vi "CopyServerCode.vi"() -> ()   [LabVIEW 2019]
uses:
  <vilib>/Utility/traverseref.llb/VI Scripting - Traverse.lvlib
  <vilib>/Utility/traverseref.llb/TRef TravTarget.ctl
  <vilib>/Utility/miscctls.llb/LVPositionTypeDef.ctl
panel:
  out "Backup path":path
  out "error out":errorcluster
  in  "Destination server name":string="gRPC1.6_Template2_server"
  in  "Source server name":string="gRPC1.6_Template_server"
  in  "target name":string="My Computer"
  in  "Project path":path=path "D:/temp test/gRPC1.6_Template.lvproj"
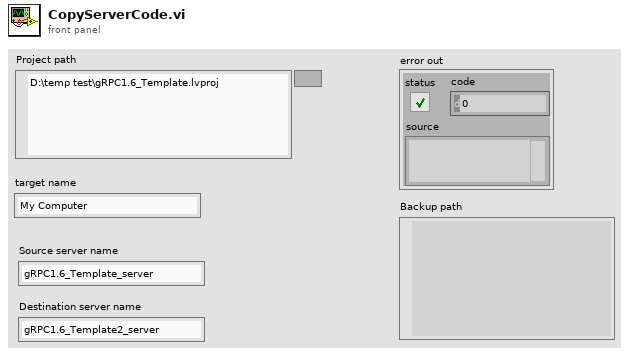
[diagram p1: front panel]
types:
  T1 = cluster{"dest":refnum<vi>, "source":refnum<vi>}[]
  T2 = cluster{"DstDiagram":refnum<vi>, "DestIndex":i32, "DstEvntStr":refnum<vi>, "SrcDiagram":refnum<vi>, "SrcIndex":i32, "SrcEvntStr":refnum<vi>}[]
  T3 = cluster{"ClassName":string, "Dest_SyncRef":refnum<vi>, "Dest_AsyncRef":refnum<vi>, "Source_SyncRef":refnum<vi>, "Source_AsyncRef":refnum<vi>}[]
  T4 = cluster{"Name":string, "DestRef":refnum<vi>, "SourceRef":refnum<vi>}[]
  T5 = cluster{string, "DestRef":refnum<vi>, refnum<vi>}
  T6 = cluster{"Name":string, "Dest_SyncRef":refnum<vi>, "Dest_AsyncRef":refnum<vi>, "Source_SyncRef":refnum<vi>, "Source_AsyncRef":refnum<vi>}
  T7 = cluster{"Name":string, "Dest_SyncRef":refnum<vi>, "Dest_AsyncRef":refnum<vi>, "Source_SyncRef":refnum<vi>, "Source_AsyncRef":refnum<vi>}[]
  T8 = typedef "TRef TravTarget.ctl" = enum16{"FP", "BD", "Other"}
  T9 = cluster{"Dest_SyncRef":refnum<vi>, "Source_SyncRef":refnum<vi>}
  T10 = cluster{"VI Ref":refnum<vi>, "VI Ref":refnum<vi>}
  T11 = cluster{"VI Ref":refnum<vi>, "VI Ref":refnum<vi>}[]
  T12 = cluster{refnum<vi>, "index of element":i32, refnum<vi>, refnum<vi>, i32, refnum<vi>}
  T13 = cluster{"DstDiagram":refnum<vi>, "index of element":i32, "DstEvntStr":refnum<vi>, "SrcDiagram":refnum<vi>, "SrcIndex":i32, "SrcEvntStr":refnum<vi>}[]
  T14 = typedef "LVPositionTypeDef.ctl" = cluster{"Left":i32, "Top":i32}
  T15 = cluster{"Src Name":string, "VI Name":string, "VI Term Name":string}[]
  T16 = cluster{"Src Name":string, "VIName":string, "Name":string}[]
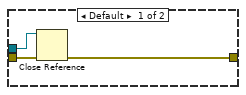
[diagram p4: hidden frame]
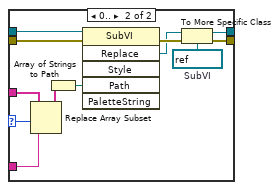
[diagram p5: hidden frame]
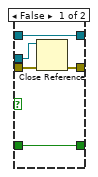
[diagram p8: hidden frame]
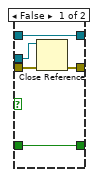
[diagram p9: hidden frame]
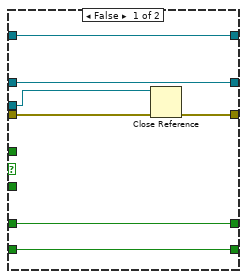
[diagram p10: hidden frame]
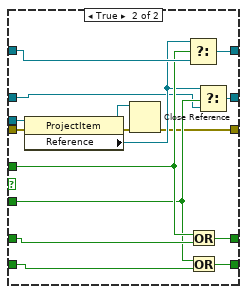
[diagram p11: hidden frame]
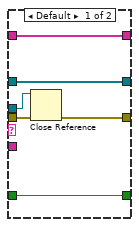
[diagram p12: hidden frame]
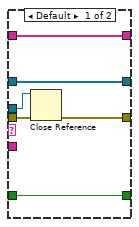
[diagram p13: hidden frame]
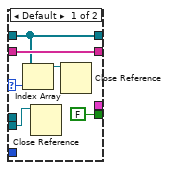
[diagram p14: hidden frame]
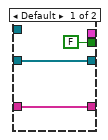
[diagram p15: hidden frame]
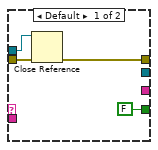
[diagram p16: hidden frame]
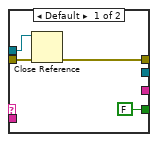
[diagram p17: hidden frame]
diagram:
  w22 = refnum<vi> refnum  # Library
  w18 = "Data Converters"
  w105 = "Backup_"
  w120 = T4 []  # CommonClasses
  w131 = string[] []  # SourceClassNames
  w129 = refnum<vi>[] []  # SourceClassPrjctRefs
  w132 = string[] []  # DestClassNames
  w136 = refnum<vi>[] []  # DestClassPrjctRefs
  w141 = refnum<vi> refnum  # Library
  w149 = refnum<vi> refnum  # Library
  w153 = ".lvlib"
  w157 = refnum<vi> refnum  # Source folder
  w158 = refnum<vi> refnum  # Dest folder
  w159 = FALSE  # found dest
  w160 = FALSE  # found source
  # "Copy destination library to source location\nand delete original destination."
  # "Verify and close project"
  # "Create Folder and add converter VIs"
  # "Add destination\nlibrary to new source\nfolder in project"
  # "Create new\nsource folder"
  # "Delete destination\nfolder\nfrom project"
  # "Delete source\ndirectory\nfrom disk"
  # "Delete source\ndirectory\nfrom project"
  # "Delete source\nlvlib from project"
  # "TODO:\nAdd check\nfor good name"
  n1 = Temporary Directory() -> (w78:path)
  n2 = Build Path(base path=w78, name or relative path=path "ServerBackups") -> (appended path=w76:path)
  n3 = Strip Path(path="Project path") -> (stripped path=w34:path)  [unwired: 1 out]
  n4 = List Folder(path=w34) -> (path out=w110:path, filenames=w139:string[], folder names=w107:string[])  [unwired: 3 in, 1 out]
  n5 = Create Folder(path (use dialog)=w76) -> (created path=w75:path)  [unwired: 2 in, 2 out]
  n6 = while {
    tunnel: w75 -> [w177]
    tunnel: [w172] -> w74
    tunnel: w105 -> [w171]
    i -> [w176]
    stop <- w173 continue-if-true
    # "Find Available\nBackup Directory"
    n7 = Number To Decimal String(number=w176) -> (decimal integer string=w174:string)  [unwired: 1 in]
    n8 = Concatenate Strings(w171, w174) -> (w175:string)
    n9 = Build Path(base path=w177, name or relative path=w175) -> (appended path=w172:path)
    n10 = call <vilib>:"Check if File or Folder Exists.vi"("path"=w172) -> ("file or folder exists?"=w173:bool)  [unwired: 8 in, 2 out]
  }
  "Backup path" <- w74
  n11 = Create Folder(path (use dialog)=w74) -> (created path=w109:path, error out=w140:errorcluster)  [unwired: 2 in, 1 out]
  n12 = for {
    shift-right: [w183] -> w108
    shift-left: w140 -> [w184]
    tunnel: w109 -> [w179]
    tunnel: w110 -> [w182]
    tunnel: w139 -> [w178] mode=indexing
    # "Backup Files"
    n13 = Build Path(base path=w182, name or relative path=w178) -> (appended path=w181:path)
    n14 = Build Path(base path=w179, name or relative path=w178) -> (appended path=w180:path)
    n15 = Copy(8:w184, 10:w180, 11:w181) -> (0:w183:errorcluster)  [unwired: 2 in, 2 out]
  }
  n16 = Concatenate Strings("^" ("string"), w105) -> (w104:string)
  n17 = for {
    shift-right: [w190] -> w7
    shift-left: w108 -> [w191]
    tunnel: w109 -> [w188]
    tunnel: w110 -> [w189]
    tunnel: w107 -> [w187] mode=indexing
    tunnel: w104 -> [w186]
    # "Backup Directories"
    n18 = Match Pattern(string=w187, regular expression=w186) -> (match substring=w185:string)  [unwired: 1 in, 3 out]
    n19 = case shown="Default" w185 {
      tunnel: w191 -> [w192 w199]
      tunnel: [w192 w198] -> w190
      tunnel: w189 -> [_ w197]
      tunnel: w188 -> [_ w194]
      tunnel: w187 -> [_ w193]
      frame "Backup_" {
        # "Don't backup\nprevious\nbackups"
      }
      frame Default {
        n20 = Build Path(base path=w197, name or relative path=w193) -> (appended path=w196:path)
        n21 = Build Path(base path=w194, name or relative path=w193) -> (appended path=w195:path)
        n22 = Copy(8:w199, 10:w195, 11:w196) -> (0:w198:errorcluster)  [unwired: 2 in, 2 out]
      }
    }
  }
  n23 = invoke class="App" method="Project.Open"(error in=w7, "Path"="Project path") -> (error out=w5:errorcluster, "Project:Open"=w6:refnum<vi>)  [unwired: 2 in, 2 out]
  n24 = invoke class="Project" method="Save"(reference=w6, error in=w5) -> (reference out=w2:refnum<vi>, error out=w3:errorcluster)  [unwired: 2 in, 2 out]
  n25 = Close Reference(reference=w2, error in (no error)=w3) -> (error out=w1:errorcluster)
  n26 = local read "Destination server name"() -> (w19:string)
  n27 = local read "Source server name"() -> (w32:string)
  n28 = Concatenate Strings(w19, ".lvlib" ("string")) -> (w27:string)
  n29 = Build Path(base path=w34, name or relative path=w32) -> (appended path=w33:path)
  n30 = Build Path(base path=w34, name or relative path=w19) -> (appended path=w26:path)
  n31 = Build Path(base path=w26, name or relative path=w27) -> (appended path=w25:path)
  n32 = Build Path(base path=w33, name or relative path=w18) -> (appended path=w31:path)
  n33 = Build Path(base path=w26, name or relative path=w18) -> (appended path=w30:path)
  n34 = call <vilib>:"Check if File or Folder Exists.vi"("error in (no error)"=w1, "path"=w31) -> ("error out"=w72:errorcluster, "file or folder exists?"=w73:bool, "dup path"=w71:path)  [unwired: 7 in]
  n35 = case shown="True" w73 {
    tunnel: w72 -> [w200 w202]
    tunnel: [w200 w204] -> w29
    tunnel: w71 -> [_ w208]
    tunnel: w30 -> [_ w203]
    tunnel: [_ w201] -> w13
    frame False {
      # "No Data Converters, do nothing"
    }
    frame True {
      # "Copy Data Converters and disconnect from Source Server Library"
      n36 = Copy(8:w202, 10:w203, 11:w208) -> (0:w207:errorcluster, 3:w205:path)  [unwired: 2 in, 1 out]
      n37 = Build Array(w205) -> (w206:path[])
      n38 = while {
        shift-right: [w215] -> _
        shift-left: w206 -> [w219]
        shift-right: [w211] -> w204
        shift-left: w207 -> [w223]
        tunnel: [w209] -> w201 mode=concatenating
        i -> [w213]
        stop <- w212 stop-if-true
        n39 = Index Array(array=w219, index=w213) -> (element=w222:path)
        n40 = List Folder(path=w222, error in=w223) -> (path out=w218:path, filenames=w220:string[], folder names=w217:string[], error out=w221:errorcluster)  [unwired: 2 in]
        n41 = for {
          shift-right: [w226] -> w211
          shift-left: w221 -> [w227]
          tunnel: w220 -> [w230] mode=indexing
          tunnel: w218 -> [w231]
          tunnel: [w225] -> w209 mode=indexing if=w224
          n42 = Build Path(base path=w231, name or relative path=w230) -> (appended path=w225:path)
          n43 = Open VI Reference(vi path=w225, error in (no error)=w227) -> (vi reference=w229:refnum<vi>, error out=w228:errorcluster)  [unwired: 4 in]
          n44 = case shown="No Error" w228 {
            selector: w228 -> [w238 _]
            tunnel: w229 -> [w239 _]
            tunnel: w227 -> [_ w240]
            tunnel: [w237 w240] -> w226
            tunnel: [TRUE _] -> w224
            frame No Error {
              n45 = invoke class="VI" method="DisconnectFromLibrary"(reference=w239, error in=w238) -> (reference out=w234:refnum<vi>, error out=w235:errorcluster)  [unwired: 1 in, 1 out]
              n46 = invoke class="VI" method="Save.Instrument"(reference=w234, error in=w235) -> (reference out=w233:refnum<vi>, error out=w236:errorcluster)  [unwired: 4 in, 4 out]
              n47 = Close Reference(reference=w233, error in (no error)=w236) -> (error out=w237:errorcluster)
            }
            frame Error {
            }
          }
        }
        n48 = for {
          tunnel: w218 -> [w243]
          tunnel: w217 -> [w242] mode=indexing
          tunnel: [w241] -> w216 mode=indexing
          n49 = Build Path(base path=w243, name or relative path=w242) -> (appended path=w241:path)
        }
        n50 = Build Array (concatenate)(w219, w216) -> (w215:path[])
        n51 = Increment(x=w213) -> (x+1=w210:i32)
        n52 = Array Size(array=w215) -> (size(s)=w214:i32)
        n53 = Less Or Equal?(x=w214, y=w210) -> (x <= y?=w212:bool)
      }
    }
  }
  n54 = invoke class="App" method="Library.Open"(error in=w29, "path"=w25) -> (error out=w24:errorcluster, "Open Library"=w23:refnum<vi>)  [unwired: 2 in, 2 out]
  n55 = To More Specific Class(target class=w22, reference=w23, error in=w24) -> (specific class reference=w20:refnum<vi>, error out=w21:errorcluster)
  n56 = invoke class="Library" method="AddItem"(reference=w20, error in=w21, "Name"=w18, "Path"=path "", "Type"="Folder") -> (reference out=w11:refnum<vi>, error out=w14:errorcluster, "AddItem"=w15:refnum<vi>)  [unwired: 1 in, 3 out]
  n57 = for {
    tunnel: w13 -> [w247] mode=indexing
    shift-right: [w245] -> _
    shift-left: w15 -> [w250]
    shift-right: [w244] -> w12
    shift-left: w14 -> [w249]
    n58 = Strip Path(path=w247) -> (name=w248:string)  [unwired: 1 out]
    n59 = invoke class="ProjectItem" method="AddItem"(reference=w250, error in=w249, "Name"=w248, "Path"=w247, "Type"="VI") -> (reference out=w245:refnum<vi>, error out=w244:errorcluster)  [unwired: 1 in, 4 out]
  }
  n60 = invoke class="Library" method="Save"(reference=w11, error in=w12) -> (reference out=w9:refnum<vi>, error out=w10:errorcluster)  [unwired: 2 in, 2 out]
  n61 = Close Reference(reference=w9, error in (no error)=w10) -> (error out=w8:errorcluster)
  n62 = invoke class="App" method="Project.Open"(error in=w8, "Path"="Project path") -> (error out=w170:errorcluster, "Project:Open"=w164:refnum<vi>)  [unwired: 2 in, 2 out]
  n63 = property class="Project"(reference=w164, error in=w170) -> (reference out=w92:refnum<vi>, error out=w168:errorcluster, "Targets"=w169:refnum<vi>[])
  n64 = for {
    tunnel: w169 -> [w261] mode=indexing
    shift-right: [w252] -> w163
    shift-left: w168 -> [w262]
    tunnel: "target name" -> [w258]
    shift-right: [w251] -> _
    shift-left: FALSE -> [w256]
    shift-right: [w254] -> w162
    shift-left: refnum<vi> refnum ("reference out") -> [w255]
    # "Get Target Item Reference"
    n65 = property class="TargetItem"(reference=w261, error in=w262) -> (reference out=w253:refnum<vi>, error out=w257:errorcluster, "Name"=w260:string)
    n66 = Equal?(x=w260, y=w258) -> (x = y?=w259:bool)
    n67 = case shown="True" w259 {
      selector: w259 -> [_ w268]
      tunnel: w257 -> [w266 w269]
      tunnel: w256 -> [w263 _]
      tunnel: w255 -> [w264 _]
      tunnel: [w264 w270] -> w254
      tunnel: w253 -> [w265 w270]
      tunnel: [w267 w269] -> w252
      tunnel: [w263 w268] -> w251
      frame False {
        n68 = Close Reference(reference=w265, error in (no error)=w266) -> (error out=w267:errorcluster)
      }
      frame True {
      }
    }
  }
  n69 = property class="TargetItem"(reference=w162, error in=w163) -> (error out=w156:errorcluster, "Children[]"=w161:refnum<vi>[])  [unwired: 1 out]
  n70 = for {
    tunnel: w161 -> [w288] mode=indexing
    shift-right: [w281] -> w152
    shift-left: w156 -> [w289]
    tunnel: "Source server name" -> [w287]
    shift-right: [w280] -> _
    shift-left: w160 -> [w285]
    shift-right: [w283] -> w151
    shift-left: w158 -> [w284]
    tunnel: "Destination server name" -> [w279]
    shift-right: [w274] -> _
    shift-left: w159 -> [w275]
    shift-right: [w272] -> w144
    shift-left: w157 -> [w273]
    # "Get Source and Destination Refs"
    n71 = property class="ProjectItem"(reference=w288, error in=w289) -> (reference out=w282:refnum<vi>, error out=w286:errorcluster, "Name"=w271:string)
    n72 = Equal?(x=w271, y=w287) -> (x = y?=w277:bool)
    n73 = Equal?(x=w271, y=w279) -> (x = y?=w276:bool)
    n74 = Or(x=w277, y=w276) -> (x .or. y?=w278:bool)
    n75 = case shown="True" w278 {
      tunnel: w286 -> [w295 w308]
      tunnel: w285 -> [w292 w299]
      tunnel: w284 -> [w293 w306]
      tunnel: [w293 w305] -> w283
      tunnel: w282 -> [w294 w303]
      tunnel: [w296 w308] -> w281
      tunnel: [w292 w302] -> w280
      tunnel: w277 -> [_ w298]
      tunnel: w276 -> [_ w297]
      tunnel: w275 -> [w291 w300]
      tunnel: [w291 w301] -> w274
      tunnel: w273 -> [w290 w307]
      tunnel: [w290 w304] -> w272
      frame False {
        n76 = Close Reference(reference=w294, error in (no error)=w295) -> (error out=w296:errorcluster)
      }
      frame True {
        n77 = Select(t=w303, s=w298, f=w307) -> (s? t:f=w304:refnum<vi>)
        n78 = Select(t=w303, s=w297, f=w306) -> (s? t:f=w305:refnum<vi>)
        n79 = Or(x=w298, y=w299) -> (x .or. y?=w302:bool)
        n80 = Or(x=w297, y=w300) -> (x .or. y?=w301:bool)
      }
    }
  }
  n81 = Concatenate Strings("Source server name", w153) -> (w142:string)
  n82 = Concatenate Strings("Destination server name", w153) -> (w143:string)
  n83 = property class="ProjectItem"(reference=w151, error in=w152) -> (reference out=w87:refnum<vi>, error out=w148:errorcluster, "Children[]"=w150:refnum<vi>[])
  n84 = for {
    tunnel: w150 -> [w319] mode=indexing
    shift-right: [w310] -> w145
    shift-left: w148 -> [w320]
    tunnel: w143 -> [w316]
    shift-right: [w309] -> _
    shift-left: FALSE -> [w314]
    shift-right: [w312] -> w37
    shift-left: w149 -> [w313]
    # "Get Dest Library Reference"
    n85 = property class="ProjectItem"(reference=w319, error in=w320) -> (reference out=w311:refnum<vi>, error out=w315:errorcluster, "Name"=w318:string)
    n86 = Equal?(x=w318, y=w316) -> (x = y?=w317:bool)
    n87 = case shown="True" w317 {
      selector: w317 -> [_ w330]
      tunnel: w315 -> [w324 w331]
      tunnel: w314 -> [w321 _]
      tunnel: w313 -> [w322 _]
      tunnel: [w322 w327] -> w312
      tunnel: w311 -> [w323 w328]
      tunnel: [w325 w329] -> w310
      tunnel: [w321 w330] -> w309
      frame False {
        n88 = Close Reference(reference=w323, error in (no error)=w324) -> (error out=w325:errorcluster)
      }
      frame True {
        w326 = refnum<vi> refnum  # Library
        n89 = To More Specific Class(target class=w326, reference=w328, error in=w331) -> (specific class reference=w327:refnum<vi>, error out=w329:errorcluster)
      }
    }
  }
  n90 = property class="ProjectItem"(reference=w144, error in=w145) -> (reference out=w94:refnum<vi>, error out=w147:errorcluster, "Children[]"=w146:refnum<vi>[])
  n91 = for {
    tunnel: w146 -> [w342] mode=indexing
    shift-right: [w333] -> w35
    shift-left: w147 -> [w343]
    tunnel: w142 -> [w339]
    shift-right: [w332] -> _
    shift-left: FALSE -> [w337]
    shift-right: [w335] -> w36
    shift-left: w141 -> [w336]
    # "Get Source Library Reference"
    n92 = property class="ProjectItem"(reference=w342, error in=w343) -> (reference out=w334:refnum<vi>, error out=w338:errorcluster, "Name"=w341:string)
    n93 = Equal?(x=w341, y=w339) -> (x = y?=w340:bool)
    n94 = case shown="True" w340 {
      selector: w340 -> [_ w353]
      tunnel: w338 -> [w347 w354]
      tunnel: w337 -> [w344 _]
      tunnel: w336 -> [w345 _]
      tunnel: [w345 w350] -> w335
      tunnel: w334 -> [w346 w351]
      tunnel: [w348 w352] -> w333
      tunnel: [w344 w353] -> w332
      frame False {
        n95 = Close Reference(reference=w346, error in (no error)=w347) -> (error out=w348:errorcluster)
      }
      frame True {
        w349 = refnum<vi> refnum  # Library
        n96 = To More Specific Class(target class=w349, reference=w351, error in=w354) -> (specific class reference=w350:refnum<vi>, error out=w352:errorcluster)
      }
    }
  }
  n97 = property class="Library"(reference=w37, error in=w35) -> (reference out=w86:refnum<vi>, error out=w138:errorcluster, "Children[]"=w137:refnum<vi>[])
  n98 = for {
    tunnel: w137 -> [w366] mode=indexing
    shift-right: [w360] -> w126
    shift-left: w138 -> [w367]
    shift-right: [w359] -> _
    shift-left: FALSE -> [w364]
    shift-right: [w362] -> w121
    shift-left: w136 -> [w363]
    shift-right: [w356] -> w122
    shift-left: w132 -> [w357]
    # "Get Dest Library Classes"
    n99 = property class="ProjectItem"(reference=w366, error in=w367) -> (reference out=w361:refnum<vi>, error out=w365:errorcluster, "Library Item Type String"=w358:string, "Name"=w355:string)
    n100 = case shown="\"LVClass\"" w358 {
      tunnel: w365 -> [w372 w382]
      tunnel: w364 -> [w369 _]
      tunnel: w363 -> [w370 w384]
      tunnel: [w370 w378] -> w362
      tunnel: w361 -> [w371 w381]
      tunnel: [w373 w383] -> w360
      tunnel: [w369 TRUE] -> w359
      tunnel: w357 -> [w368 w376]
      tunnel: [w368 w375] -> w356
      tunnel: w355 -> [_ w374]
      frame Default {
        n101 = Close Reference(reference=w371, error in (no error)=w372) -> (error out=w373:errorcluster)
      }
      frame "LVClass" {
        w380 = refnum<vi> refnum  # LVClassLibrary
        n102 = To More Specific Class(target class=w380, reference=w381, error in=w382) -> (specific class reference=w379:refnum<vi>, error out=w383:errorcluster)
        n103 = Build Array (concatenate)(w376, w374) -> (w375:string[])
        n104 = Build Array (concatenate)(w384, w379) -> (w378:refnum<vi>[])
      }
    }
  }
  n105 = property class="Library"(reference=w36, error in=w126) -> (reference out=w95:refnum<vi>, error out=w127:errorcluster, "Children[]"=w128:refnum<vi>[])
  n106 = for {
    tunnel: w128 -> [w396] mode=indexing
    shift-right: [w390] -> w123
    shift-left: w127 -> [w397]
    shift-right: [w389] -> _
    shift-left: FALSE -> [w394]
    shift-right: [w392] -> w124
    shift-left: w129 -> [w393]
    shift-right: [w386] -> w125
    shift-left: w131 -> [w387]
    # "Get Source Library Classes"
    n107 = property class="ProjectItem"(reference=w396, error in=w397) -> (reference out=w391:refnum<vi>, error out=w395:errorcluster, "Library Item Type String"=w388:string, "Name"=w385:string)
    n108 = case shown="\"LVClass\"" w388 {
      tunnel: w395 -> [w402 w412]
      tunnel: w394 -> [w399 _]
      tunnel: w393 -> [w400 w414]
      tunnel: [w400 w409] -> w392
      tunnel: w391 -> [w401 w411]
      tunnel: [w403 w413] -> w390
      tunnel: [w399 TRUE] -> w389
      tunnel: w387 -> [w398 w407]
      tunnel: [w398 w406] -> w386
      tunnel: w385 -> [_ w405]
      frame Default {
        n109 = Close Reference(reference=w401, error in (no error)=w402) -> (error out=w403:errorcluster)
      }
      frame "LVClass" {
        w404 = refnum<vi> refnum  # LVClassLibrary
        n110 = To More Specific Class(target class=w404, reference=w411, error in=w412) -> (specific class reference=w410:refnum<vi>, error out=w413:errorcluster)
        n111 = Build Array (concatenate)(w407, w405) -> (w406:string[])
        n112 = Build Array (concatenate)(w414, w410) -> (w409:refnum<vi>[])
      }
    }
  }
  n113 = for {
    tunnel: w125 -> [w421] mode=indexing
    tunnel: w124 -> [w422] mode=indexing
    shift-right: [w424] -> w117
    shift-left: w123 -> [w425]
    shift-right: [w416] -> _
    shift-left: w122 -> [w419]
    shift-right: [w415] -> _
    shift-left: w121 -> [w420]
    shift-right: [w417] -> w118
    shift-left: w120 -> [w418]
    shift-right: [w423] -> _
    shift-left: FALSE -> [w427]
    # "Find Common Classes"
    n114 = Search 1D Array(1D array=w419, element=w421) -> (index of element=w426:i32)  [unwired: 1 in]
    n115 = case shown="Default" w426 {
      selector: w426 -> [w436 _]
      tunnel: w427 -> [_ w442]
      tunnel: w425 -> [w437 w443]
      tunnel: [w437 w443] -> w424
      tunnel: [TRUE w442] -> w423
      tunnel: w422 -> [w428 _]
      tunnel: w421 -> [w435 _]
      tunnel: w420 -> [w431 w439]
      tunnel: w419 -> [w430 w440]
      tunnel: w418 -> [w433 w441]
      tunnel: [w429 w441] -> w417
      tunnel: [w430 w440] -> w416
      tunnel: [w431 w439] -> w415
      frame Default {
        n116 = Index Array(array=w431, index=w436) -> (element=w434:refnum<vi>)
        n117 = Bundle(w435, "DestRef"=w434, w428) -> (w432:T5)  [unwired: 1 in]
        n118 = Build Array (concatenate)(w433, w432) -> (w429:T4)
      }
      frame ..-1 {
      }
    }
  }
  n119 = for {
    tunnel: w118 -> [w486] mode=indexing
    shift-right: [w462] -> w102
    shift-left: T3 [] -> [w464]
    shift-right: [w444] -> w115
    shift-left: w117 -> [w457]
    w445 = "Server API" ("target name 2")
    w477 = refnum<vi> refnum  # Dest_AsyncRef
    w476 = refnum<vi> refnum  # Dest_SyncRef
    w478 = refnum<vi> refnum  # Source_AsyncRef
    w479 = refnum<vi> refnum  # Source_SyncRef
    # "Find Sync and ASync VI refs"
    n120 = Unbundle By Name(w486) -> ("Name"=w469:string, "DestRef"=w449:refnum<vi>, "SourceRef"=w456:refnum<vi>)
    n121 = property class="LVClassLibrary"(reference=w456, error in=w457) -> (error out=w460:errorcluster, "Children[]"=w461:refnum<vi>[])  [unwired: 1 out]
    n122 = for {
      tunnel: w461 -> [w517] mode=indexing
      shift-right: [w508] -> w454
      shift-left: w460 -> [w518]
      tunnel: w445 -> [w514]
      shift-right: [w507] -> _
      shift-left: FALSE -> [w512]
      shift-right: [w510] -> w455
      shift-left: refnum<vi> refnum ("reference out") -> [w511]
      # "Find Server API Folder"
      n123 = property class="ProjectItem"(reference=w517, error in=w518) -> (reference out=w509:refnum<vi>, error out=w513:errorcluster, "Name"=w516:string)
      n124 = Equal?(x=w516, y=w514) -> (x = y?=w515:bool)
      n125 = case shown="True" w515 {
        selector: w515 -> [_ w524]
        tunnel: w513 -> [w522 w525]
        tunnel: w512 -> [w519 _]
        tunnel: w511 -> [w520 _]
        tunnel: [w520 w526] -> w510
        tunnel: w509 -> [w521 w526]
        tunnel: [w523 w525] -> w508
        tunnel: [w519 w524] -> w507
        frame False {
          n126 = Close Reference(reference=w521, error in (no error)=w522) -> (error out=w523:errorcluster)
        }
        frame True {
        }
      }
    }
    n127 = property class="ProjectItem"(reference=w455, error in=w454) -> (error out=w485:errorcluster, "Children[]"=w484:refnum<vi>[])  [unwired: 1 out]
    n128 = for {
      tunnel: w484 -> [w586] mode=indexing
      shift-right: [w579] -> w446
      shift-left: w485 -> [w587]
      tunnel: "Start Sync.vi" ("Source server name") -> [w585]
      shift-right: [w578] -> _
      shift-left: FALSE -> [w583]
      shift-right: [w581] -> w465
      shift-left: w478 -> [w582]
      tunnel: "Start Async.vi" ("Destination server name") -> [w577]
      shift-right: [w572] -> _
      shift-left: FALSE -> [w573]
      shift-right: [w570] -> w466
      shift-left: w479 -> [w571]
      # "Get Sync and Async VI Refs"
      n129 = property class="ProjectItem"(reference=w586, error in=w587) -> (reference out=w580:refnum<vi>, error out=w584:errorcluster, "Name"=w569:string)
      n130 = Equal?(x=w569, y=w585) -> (x = y?=w575:bool)
      n131 = Equal?(x=w569, y=w577) -> (x = y?=w574:bool)
      n132 = Or(x=w575, y=w574) -> (x .or. y?=w576:bool)
      n133 = case shown="False" w576 {
        tunnel: w584 -> [w593 w601]
        tunnel: w583 -> [w590 w604]
        tunnel: w582 -> [w591 w595]
        tunnel: [w591 w609] -> w581
        tunnel: w580 -> [w592 w600]
        tunnel: [w594 w596] -> w579
        tunnel: [w590 w607] -> w578
        tunnel: w575 -> [_ w603]
        tunnel: w574 -> [_ w602]
        tunnel: w573 -> [w589 w605]
        tunnel: [w589 w606] -> w572
        tunnel: w571 -> [w588 w610]
        tunnel: [w588 w608] -> w570
        frame False {
          n134 = Close Reference(reference=w592, error in (no error)=w593) -> (error out=w594:errorcluster)
        }
        frame True {
          n135 = property class="ProjectItem"(reference=w600, error in=w601) -> (reference out=w597:refnum<vi>, error out=w598:errorcluster, "Reference"=w599:refnum<vi>)
          n136 = Close Reference(reference=w597, error in (no error)=w598) -> (error out=w596:errorcluster)
          n137 = Select(t=w599, s=w603, f=w610) -> (s? t:f=w608:refnum<vi>)
          n138 = Or(x=w603, y=w604) -> (x .or. y?=w607:bool)
          n139 = Or(x=w602, y=w605) -> (x .or. y?=w606:bool)
          n140 = Select(t=w599, s=w602, f=w595) -> (s? t:f=w609:refnum<vi>)
        }
      }
    }
    n141 = property class="LVClassLibrary"(reference=w449, error in=w446) -> (error out=w451:errorcluster, "Children[]"=w450:refnum<vi>[])  [unwired: 1 out]
    n142 = for {
      tunnel: w450 -> [w497] mode=indexing
      shift-right: [w488] -> w448
      shift-left: w451 -> [w498]
      tunnel: w445 -> [w494]
      shift-right: [w487] -> _
      shift-left: FALSE -> [w492]
      shift-right: [w490] -> w447
      shift-left: refnum<vi> refnum ("reference out") -> [w491]
      # "Find Server API Folder"
      n143 = property class="ProjectItem"(reference=w497, error in=w498) -> (reference out=w489:refnum<vi>, error out=w493:errorcluster, "Name"=w496:string)
      n144 = Equal?(x=w496, y=w494) -> (x = y?=w495:bool)
      n145 = case shown="True" w495 {
        selector: w495 -> [_ w504]
        tunnel: w493 -> [w502 w505]
        tunnel: w492 -> [w499 _]
        tunnel: w491 -> [w500 _]
        tunnel: [w500 w506] -> w490
        tunnel: w489 -> [w501 w506]
        tunnel: [w503 w505] -> w488
        tunnel: [w499 w504] -> w487
        frame False {
          n146 = Close Reference(reference=w501, error in (no error)=w502) -> (error out=w503:errorcluster)
        }
        frame True {
        }
      }
    }
    n147 = property class="ProjectItem"(reference=w447, error in=w448) -> (error out=w470:errorcluster, "Children[]"=w471:refnum<vi>[])  [unwired: 1 out]
    n148 = for {
      tunnel: w471 -> [w544] mode=indexing
      shift-right: [w537] -> w444
      shift-left: w470 -> [w545]
      tunnel: "Start Sync.vi" ("Source server name") -> [w543]
      shift-right: [w536] -> _
      shift-left: FALSE -> [w541]
      shift-right: [w539] -> w467
      shift-left: w477 -> [w540]
      tunnel: "Start Async.vi" ("Destination server name") -> [w535]
      shift-right: [w530] -> _
      shift-left: FALSE -> [w531]
      shift-right: [w528] -> w468
      shift-left: w476 -> [w529]
      # "Get Sync and Async VI Refs"
      n149 = property class="ProjectItem"(reference=w544, error in=w545) -> (reference out=w538:refnum<vi>, error out=w542:errorcluster, "Name"=w527:string)
      n150 = Equal?(x=w527, y=w543) -> (x = y?=w533:bool)
      n151 = Equal?(x=w527, y=w535) -> (x = y?=w532:bool)
      n152 = Or(x=w533, y=w532) -> (x .or. y?=w534:bool)
      n153 = case shown="True" w534 {
        tunnel: w542 -> [w551 w559]
        tunnel: w541 -> [w548 w562]
        tunnel: w540 -> [w549 w556]
        tunnel: [w549 w567] -> w539
        tunnel: w538 -> [w550 w558]
        tunnel: [w552 w555] -> w537
        tunnel: [w548 w565] -> w536
        tunnel: w533 -> [_ w561]
        tunnel: w532 -> [_ w560]
        tunnel: w531 -> [w547 w563]
        tunnel: [w547 w564] -> w530
        tunnel: w529 -> [w546 w568]
        tunnel: [w546 w566] -> w528
        frame False {
          n154 = Close Reference(reference=w550, error in (no error)=w551) -> (error out=w552:errorcluster)
        }
        frame True {
          n155 = property class="ProjectItem"(reference=w558, error in=w559) -> (reference out=w553:refnum<vi>, error out=w554:errorcluster, "Reference"=w557:refnum<vi>)
          n156 = Close Reference(reference=w553, error in (no error)=w554) -> (error out=w555:errorcluster)
          n157 = Select(t=w557, s=w561, f=w568) -> (s? t:f=w566:refnum<vi>)
          n158 = Or(x=w561, y=w562) -> (x .or. y?=w565:bool)
          n159 = Or(x=w560, y=w563) -> (x .or. y?=w564:bool)
          n160 = Select(t=w557, s=w560, f=w556) -> (s? t:f=w567:refnum<vi>)
        }
      }
    }
    n161 = Bundle("Name"=w469, "Dest_SyncRef"=w468, "Dest_AsyncRef"=w467, "Source_SyncRef"=w466, "Source_AsyncRef"=w465) -> (w463:T6)  [unwired: 1 in]
    n162 = Build Array (concatenate)(w464, w463) -> (w462:T7)
  }
  n163 = for {
    tunnel: w102 -> [w635] mode=indexing
    shift-right: [w612] -> w112
    shift-left: w115 -> [w624]
    shift-right: [w611] -> w97
    shift-left: T1 [] -> [w617]
    # "Find Destination and Source VIs"
    n164 = Unbundle By Name(w635) -> ("Dest_SyncRef"=w619:refnum<vi>, "Dest_AsyncRef"=w625:refnum<vi>, "Source_SyncRef"=w618:refnum<vi>, "Source_AsyncRef"=w634:refnum<vi>)
    n165 = call <vilib>:"Traverse for GObjects.vi"("Traverse Target"=TRef_TravTarget."BD", "error in (no error)"=w624, "Class Name"="SubVI", "VI Refnum"=w634) -> ("error out"=w630:errorcluster, "References"=w631:refnum<vi>[])  [unwired: 4 in, 2 out]
    n166 = for {
      tunnel: w631 -> [w696] mode=indexing
      tunnel: [w688] -> w621 mode=indexing if=w685
      tunnel: [w687] -> w620 mode=indexing if=w685
      shift-right: [w686] -> w614
      shift-left: w630 -> [w698]
      w697 = refnum<vi> refnum  # SubVI
      # "Get Source Async Command VIs List"
      n167 = To More Specific Class(target class=w697, reference=w696, error in=w698) -> (specific class reference=w694:refnum<vi>, error out=w695:errorcluster)
      n168 = property class="SubVI"(reference=w694, error in=w695) -> (reference out=w690:refnum<vi>, error out=w691:errorcluster, "VIName"=w689:string)
      n169 = Match Pattern(string=w689, regular expression="RPC Method") -> (match substring=w692:string, after substring=w684:string)  [unwired: 1 in, 2 out]
      n170 = case shown="\"RPC Method\"" w692 {
        selector: w692 -> [_ w705]
        tunnel: w691 -> [w702 w712]
        tunnel: w690 -> [w701 w711]
        tunnel: [w700 w708] -> w686
        tunnel: [_ w707] -> w688
        tunnel: [_ w703] -> w687
        tunnel: [FALSE TRUE] -> w685
        tunnel: w684 -> [_ w704]
        frame Default {
          n171 = Close Reference(reference=w701, error in (no error)=w702) -> (error out=w700:errorcluster)
        }
        frame "RPC Method" {
          n172 = property class="SubVI"(reference=w711, error in=w712) -> (reference out=w709:refnum<vi>, error out=w710:errorcluster, "VI Ref"=w707:refnum<vi>)
          n173 = Concatenate Strings(w705, w704) -> (w703:string)
          n174 = Close Reference(reference=w709, error in (no error)=w710) -> (error out=w708:errorcluster)
        }
      }
    }
    n175 = call <vilib>:"Traverse for GObjects.vi"("Traverse Target"=TRef_TravTarget."BD", "error in (no error)"=w624, "Class Name"="SubVI", "VI Refnum"=w625) -> ("error out"=w629:errorcluster, "References"=w628:refnum<vi>[])  [unwired: 4 in, 2 out]
    n176 = Bundle("Dest_SyncRef"=w619, "Source_SyncRef"=w618) -> (w616:T9)  [unwired: 1 in]
    n177 = for {
      tunnel: w628 -> [w667] mode=indexing
      tunnel: [w659] -> w623 mode=indexing if=w656
      tunnel: [w658] -> w622 mode=indexing if=w656
      shift-right: [w657] -> w613
      shift-left: w629 -> [w669]
      w668 = refnum<vi> refnum  # SubVI
      # "Get Destination Async Command VIs List"
      n178 = To More Specific Class(target class=w668, reference=w667, error in=w669) -> (specific class reference=w665:refnum<vi>, error out=w666:errorcluster)
      n179 = property class="SubVI"(reference=w665, error in=w666) -> (reference out=w661:refnum<vi>, error out=w662:errorcluster, "VIName"=w660:string)
      n180 = Match Pattern(string=w660, regular expression="RPC Method") -> (match substring=w663:string, after substring=w655:string)  [unwired: 1 in, 2 out]
      n181 = case shown="\"RPC Method\"" w663 {
        selector: w663 -> [_ w676]
        tunnel: w662 -> [w673 w683]
        tunnel: w661 -> [w672 w682]
        tunnel: [w671 w679] -> w657
        tunnel: [_ w678] -> w659
        tunnel: [_ w674] -> w658
        tunnel: [FALSE TRUE] -> w656
        tunnel: w655 -> [_ w675]
        frame Default {
          n182 = Close Reference(reference=w672, error in (no error)=w673) -> (error out=w671:errorcluster)
        }
        frame "RPC Method" {
          n183 = property class="SubVI"(reference=w682, error in=w683) -> (reference out=w680:refnum<vi>, error out=w681:errorcluster, "VI Ref"=w678:refnum<vi>)
          n184 = Concatenate Strings(w676, w675) -> (w674:string)
          n185 = Close Reference(reference=w680, error in (no error)=w681) -> (error out=w679:errorcluster)
        }
      }
    }
    n186 = for {
      tunnel: w623 -> [w642] mode=indexing
      tunnel: w622 -> [w644] mode=indexing
      shift-right: [w641] -> _
      shift-left: w621 -> [w640]
      shift-right: [w639] -> _
      shift-left: w620 -> [w638]
      tunnel: [w637] -> w615 mode=indexing if=w636
      # "Construct Dest/Source VI Pairs"
      n187 = Search 1D Array(1D array=w638, element=w644) -> (index of element=w643:i32)  [unwired: 1 in]
      n188 = case shown="0.." w643 {
        selector: w643 -> [_ w652]
        tunnel: w642 -> [_ w651]
        tunnel: [w647 w653] -> w641
        tunnel: w640 -> [w647 w653]
        tunnel: [w646 w654] -> w639
        tunnel: w638 -> [w646 w654]
        tunnel: [_ w649] -> w637
        tunnel: [FALSE TRUE] -> w636
        frame Default {
        }
        frame 0.. {
          n189 = Index Array(array=w653, index=w652) -> (element=w650:refnum<vi>)
          n190 = Bundle("VI Ref"=w651, "VI Ref"=w650) -> (w649:T10)  [unwired: 1 in]
        }
      }
    }
    n191 = Merge Errors(w613, w614) -> (w612:errorcluster)
    n192 = Build Array (concatenate)(w617, w616, w615) -> (w611:T11)
  }
  n193 = for {
    shift-right: [w715] -> w98
    shift-left: T2 [] -> [w717]
    tunnel: w97 -> [w742] mode=indexing
    shift-right: [w718] -> w111
    shift-left: w112 -> [w735]
    w729 = refnum<vi> refnum  # EventStructure
    w734 = refnum<vi> refnum  # EventStructure
    # "Find Destination and Source Diagrams"
    n194 = Unbundle By Name(w742) -> ("dest"=w737:refnum<vi>, "source"=w736:refnum<vi>)
    n195 = call <vilib>:"Traverse for GObjects.vi"("Traverse Target"=TRef_TravTarget."BD", "error in (no error)"=w735, "Class Name"="EventStructure", "VI Refnum"=w736) -> ("error out"=w741:errorcluster, "References"=w726:refnum<vi>[])  [unwired: 4 in, 2 out]
    n196 = call <vilib>:"Traverse for GObjects.vi"("Traverse Target"=TRef_TravTarget."BD", "error in (no error)"=w735, "Class Name"="EventStructure", "VI Refnum"=w737) -> ("error out"=w740:errorcluster, "References"=w731:refnum<vi>[])  [unwired: 4 in, 2 out]
    n197 = Index Array(array=w726) -> (element=w725:refnum<vi>)  [unwired: 1 in]
    n198 = Index Array(array=w731) -> (element=w730:refnum<vi>)  [unwired: 1 in]
    n199 = To More Specific Class(target class=w729, reference=w725, error in=w741) -> (specific class reference=w727:refnum<vi>, error out=w728:errorcluster)
    n200 = To More Specific Class(target class=w734, reference=w730, error in=w740) -> (specific class reference=w732:refnum<vi>, error out=w733:errorcluster)
    n201 = property class="EvntStruct"(reference=w727, error in=w728) -> (reference out=w714:refnum<vi>, error out=w720:errorcluster, "Frames[]"=w722:refnum<vi>[], "EventSelectors"=w721:string[])
    n202 = property class="EvntStruct"(reference=w732, error in=w733) -> (reference out=w713:refnum<vi>, error out=w719:errorcluster, "Frames[]"=w724:refnum<vi>[], "EventSelectors"=w723:string[])
    n203 = Merge Errors(w719, w720) -> (w718:errorcluster)
    n204 = for {
      tunnel: w722 -> [w748] mode=indexing
      tunnel: w721 -> [w756] mode=indexing
      shift-right: [w752] -> _
      shift-left: w724 -> [w751]
      shift-right: [w754] -> _
      shift-left: w723 -> [w753]
      tunnel: [w750] -> w716 mode=indexing if=w749
      tunnel: w714 -> [w746]
      tunnel: w713 -> [w745]
      i -> [w747]
      # "Match diagram names"
      n205 = Search 1D Array(1D array=w753, element=w756) -> (index of element=w755:i32)  [unwired: 1 in]
      n206 = case shown="0.." w755 {
        selector: w755 -> [w759 w765]
        tunnel: w748 -> [w760 w770]
        tunnel: [w761 w772] -> w754
        tunnel: w753 -> [w761 w772]
        tunnel: [w758 w771] -> w752
        tunnel: w751 -> [w758 w771]
        tunnel: [_ w768] -> w750
        tunnel: [FALSE TRUE] -> w749
        tunnel: w747 -> [_ w766]
        tunnel: w746 -> [_ w764]
        tunnel: w745 -> [_ w763]
        frame Default {
          n207 = Index Array(array=w758, index=w759) -> (element=w757:refnum<vi>)
          n208 = Close Reference(reference=w760) -> ()  [unwired: 1 in, 1 out]
          n209 = Close Reference(reference=w757) -> ()  [unwired: 1 in, 1 out]
        }
        frame 0.. {
          n210 = Index Array(array=w771, index=w765) -> (element=w769:refnum<vi>)
          n211 = Bundle(w769, "index of element"=w765, w763, w770, w766, w764) -> (w768:T12)  [unwired: 1 in]
        }
      }
    }
    n212 = Build Array (concatenate)(w717, w716) -> (w715:T13)
  }
  n213 = local read "Destination server name"() -> (w69:string)
  n214 = local read "Source server name"() -> (w70:string)
  n215 = for {
    tunnel: [w821] -> _ mode=indexing
    tunnel: w98 -> [w821] mode=indexing
    shift-right: [w783] -> w103
    shift-left: w111 -> [w812]
    tunnel: w70 -> [w774]
    tunnel: w69 -> [w775]
    # "Copy code and rewire"
    n216 = Unbundle By Name(w821) -> ("DstEvntStr"=w796:refnum<vi>, "DestIndex"=w795:i32, "DstDiagram"=w779:refnum<vi>, "SrcEvntStr"=w800:refnum<vi>, "SrcIndex"=w799:i32, "SrcDiagram"=w820:refnum<vi>)
    n217 = property class="Diag"(reference=w820, error in=w812) -> (error out=w819:errorcluster, "OwningVI"=w818:refnum<vi>, "AllObjs[]"=w815:refnum<vi>[], "Wires[]"=w810:refnum<vi>[])  [unwired: 1 out]
    n218 = property class="VI"(reference=w818, error in=w819) -> (reference out=w778:refnum<vi>, error out=w816:errorcluster, "Diagram"=w817:refnum<vi>)
    n219 = Build Array (concatenate)(w815, w810) -> (w811:refnum<vi>[])
    n220 = invoke class="TopLvlDiag" method="Make Selection"(reference=w817, error in=w816, "Objects"=w811) -> (reference out=w813:refnum<vi>, error out=w814:errorcluster)  [unwired: 1 in, 2 out]
    n221 = invoke class="TopLvlDiag" method="Copy Selection"(reference=w813, error in=w814) -> (error out=w809:errorcluster)  [unwired: 1 in, 2 out]
    n222 = invoke class="EvntStruct" method="GetEventDataNode"(reference=w800, error in=w809, "frameIndex"=w799) -> (error out=w807:errorcluster, "GetEventDataNode"=w808:refnum<vi>)  [unwired: 1 in, 2 out]
    n223 = property class="NmdUnbndl"(reference=w808, error in=w807) -> (error out=w806:errorcluster, "OutputTerms[]"=w805:refnum<vi>[], "ElemNms[]"=w804:string[])  [unwired: 1 out]
    n224 = for {
      shift-right: [w883] -> w803
      shift-left: w806 -> [w878]
      tunnel: w805 -> [w886] mode=indexing
      tunnel: w804 -> [w885] mode=indexing
      shift-right: [w881] -> w784
      shift-left: T15 [] -> [w882]
      i -> [w880]
      # "Find data connections"
      n225 = property class="Term"(reference=w886, error in=w878) -> (error out=w879:errorcluster, "Wire.Terms[]"=w884:refnum<vi>[])  [unwired: 1 out]
      n226 = case shown="No Error" w879 {
        tunnel: w885 -> [_ w891]
        tunnel: w884 -> [_ w892]
        tunnel: [w887 w893] -> w883
        tunnel: w882 -> [w888 w890]
        tunnel: [w888 w889] -> w881
        tunnel: w880 -> [_ _]
        tunnel: w878 -> [w887 _]
        frame Error {
          # "Error means no wire connected"
        }
        frame No Error {
          # "Terminal is wired - find other end of wire"
          n227 = for {
            shift-right: [w899] -> w893
            shift-left: _ -> [w905]
            tunnel: w892 -> [w904] mode=indexing
            tunnel: w891 -> [w894]
            shift-right: [w896] -> w889
            shift-left: w890 -> [w897]
            w903 = refnum<vi> refnum  # SubVI
            n228 = property class="Term"(reference=w904, error in=w905) -> (error out=w900:errorcluster, "Owner"=w902:refnum<vi>, "Name"=w895:string)  [unwired: 1 out]
            n229 = To More Specific Class(target class=w903, reference=w902, error in=w900) -> (specific class reference=w898:refnum<vi>, error out=w901:errorcluster)
            n230 = case shown="No Error" w901 {
              selector: w901 -> [w913 _]
              tunnel: w900 -> [_ w916]
              tunnel: [w906 w916] -> w899
              tunnel: w898 -> [w914 _]
              tunnel: w897 -> [w908 w915]
              tunnel: [w907 w915] -> w896
              tunnel: w894 -> [w912 _]
              tunnel: w895 -> [w910 _]
              frame No Error {
                n231 = property class="SubVI"(reference=w914, error in=w913) -> (error out=w906:errorcluster, "VIName"=w911:string)  [unwired: 1 out]
                n232 = Bundle(w912, "VIName"=w911, "Name"=w910) -> (w909:cluster{string, "VIName":string, "Name":string})  [unwired: 1 in]
                n233 = Build Array (concatenate)(w908, w909) -> (w907:T16)
              }
              frame Error {
              }
            }
          }
        }
      }
    }
    n234 = invoke class="Diag" method="Paste"(reference=w779, error in=w803, "Pos"=T14 {"Left"=100, "Top"=100} ("Position")) -> (error out=w794:errorcluster)  [unwired: 1 in, 3 out]
    n235 = call <vilib>:"Traverse for GObjects.vi"("Other Refnum"=w779, "Traverse Target"=TRef_TravTarget."Other", "error in (no error)"=w794, "Class Name"="SubVI", "VI Refnum"=w778) -> ("error out"=w791:errorcluster, "References"=w790:refnum<vi>[])  [unwired: 3 in, 2 out]
    n236 = for {
      tunnel: w790 -> [w861] mode=indexing
      shift-right: [w849] -> w780
      shift-left: w791 -> [w862]
      tunnel: [w850] -> w787 mode=indexing
      tunnel: [w858] -> w786 mode=indexing
      tunnel: w774 -> [w856]
      tunnel: w775 -> [w854]
      w863 = refnum<vi> refnum  # SubVI
      # "Get names and replace old library VIs with new library code"
      n237 = To More Specific Class(target class=w863, reference=w861, error in=w862) -> (specific class reference=w860:refnum<vi>, error out=w859:errorcluster)
      n238 = property class="SubVI"(reference=w860, error in=w859) -> (reference out=w853:refnum<vi>, error out=w852:errorcluster, "VIName"=w858:string, "VIPath"=w857:path)
      n239 = Path to Array of Strings(0:w857) -> (2:w855:string[])  [unwired: 1 out]
      n240 = Search 1D Array(1D array=w855, element=w856) -> (index of element=w851:i32)  [unwired: 1 in]
      n241 = case shown="Default" w851 {
        selector: w851 -> [_ w871]
        tunnel: w855 -> [_ w877]
        tunnel: w854 -> [_ w876]
        tunnel: w853 -> [w865 w874]
        tunnel: w852 -> [w864 w873]
        tunnel: [w865 w866] -> w850
        tunnel: [w864 w870] -> w849
        frame Default {
        }
        frame 0.. {
          w867 = refnum<vi> refnum  # SubVI
          n242 = Replace Array Subset(array=w877, new element=w876, index=w871) -> (w875:string[])
          n243 = Array of Strings to Path(0:w875) -> (2:w872:path)  [unwired: 1 in]
          n244 = invoke class="SubVI" method="Replace"(reference=w874, error in=w873, "Path"=w872) -> (error out=w869:errorcluster, "Replace"=w868:refnum<vi>)  [unwired: 3 in, 4 out]
          n245 = To More Specific Class(target class=w867, reference=w868, error in=w869) -> (specific class reference=w866:refnum<vi>, error out=w870:errorcluster)
        }
      }
    }
    n246 = call <vilib>:"Traverse for GObjects.vi"("Other Refnum"=w779, "Traverse Target"=TRef_TravTarget."Other", "error in (no error)"=w780, "Class Name"="ClusterConstant", "VI Refnum"=w778) -> ("error out"=w776:errorcluster, "References"=w773:refnum<vi>[])  [unwired: 3 in, 2 out]
    n247 = for {
      tunnel: w773 -> [w833] mode=indexing
      shift-right: [w824] -> w777
      shift-left: w776 -> [w834]
      tunnel: w774 -> [w830]
      tunnel: w775 -> [w828]
      w835 = refnum<vi> refnum  # ClusterConstant
      # "Replace old library typedefs with new library code"
      n248 = To More Specific Class(target class=w835, reference=w833, error in=w834) -> (specific class reference=w832:refnum<vi>, error out=w831:errorcluster)
      n249 = property class="ClustCnst"(reference=w832, error in=w831) -> (reference out=w827:refnum<vi>, error out=w826:errorcluster, "DependPaths"=w823:path[])
      n250 = Index Array(array=w823) -> (element=w822:path)  [unwired: 1 in]
      n251 = Path to Array of Strings(0:w822) -> (2:w829:string[])  [unwired: 1 out]
      n252 = Search 1D Array(1D array=w829, element=w830) -> (index of element=w825:i32)  [unwired: 1 in]
      n253 = case shown="0.." w825 {
        selector: w825 -> [_ w842]
        tunnel: w829 -> [_ w848]
        tunnel: w828 -> [_ w847]
        tunnel: w827 -> [w836 w845]
        tunnel: w826 -> [w838 w844]
        tunnel: [w837 w841] -> w824
        frame Default {
          n254 = Close Reference(reference=w836, error in (no error)=w838) -> (error out=w837:errorcluster)
        }
        frame 0.. {
          n255 = Replace Array Subset(array=w848, new element=w847, index=w842) -> (w846:string[])
          n256 = Array of Strings to Path(0:w846) -> (2:w843:path)  [unwired: 1 in]
          n257 = invoke class="ClustCnst" method="Replace"(reference=w845, error in=w844, "Path"=w843) -> (error out=w839:errorcluster, "Replace"=w840:refnum<vi>)  [unwired: 3 in, 4 out]
          n258 = Close Reference(reference=w840, error in (no error)=w839) -> (error out=w841:errorcluster)
        }
      }
    }
    n259 = invoke class="EvntStruct" method="GetEventDataNode"(reference=w796, error in=w777, "frameIndex"=w795) -> (error out=w797:errorcluster, "GetEventDataNode"=w798:refnum<vi>)  [unwired: 1 in, 2 out]
    n260 = property class="NmdUnbndl"(reference=w798, error in=w797) -> (error out=w785:errorcluster, "OutputTerms[]"=w788:refnum<vi>[], "ElemNms[]"=w789:string[])  [unwired: 1 out]
    n261 = for {
      shift-right: [w931] -> _
      shift-left: w787 -> [w931]
      shift-right: [w934] -> _
      shift-left: w786 -> [w934]
      shift-right: [w922] -> w783
      shift-left: w785 -> [w930]
      tunnel: w784 -> [w935] mode=indexing
      shift-right: [w918] -> _
      shift-left: w788 -> [w918]
      shift-right: [w921] -> _
      shift-left: w789 -> [w921]
      # "Wire to data block"
      n262 = Unbundle By Name(w935) -> ("VI Name"=w933:string, "VI Term Name"=w926:string, "Src Name"=w920:string)
      n263 = Search 1D Array(1D array=w921, element=w920) -> (index of element=w919:i32)  [unwired: 1 in]
      n264 = Index Array(array=w918, index=w919) -> (element=w917:refnum<vi>)
      n265 = Search 1D Array(1D array=w934, element=w933) -> (index of element=w932:i32)  [unwired: 1 in]
      n266 = Index Array(array=w931, index=w932) -> (element=w929:refnum<vi>)
      n267 = property class="SubVI"(reference=w929, error in=w930) -> (error out=w927:errorcluster, "Terms[]"=w928:refnum<vi>[])  [unwired: 1 out]
      n268 = for {
        tunnel: w928 -> [w941] mode=indexing
        shift-right: [w936] -> w924
        shift-left: w927 -> [w942]
        tunnel: w926 -> [w939]
        tunnel: [w937] -> w925
        stop <- w938 stop-if-true
        n269 = property class="Term"(reference=w941, error in=w942) -> (reference out=w937:refnum<vi>, error out=w936:errorcluster, "Name"=w940:string)
        n270 = Equal?(x=w940, y=w939) -> (x = y?=w938:bool)
      }
      n271 = invoke class="Term" method="Connect Wire"(reference=w925, error in=w924, "Wire Source"=w917, "Auto Route? (F)"=TRUE) -> (error out=w922:errorcluster)  [unwired: 3 in, 6 out]
    }
  }
  n272 = for {
    shift-right: [w944] -> w101
    shift-left: w103 -> [w945]
    tunnel: w97 -> [w943] mode=indexing
    tunnel: [w943] -> w99 mode=indexing
    # "Clean up bad wires"
    n273 = Unbundle By Name(w943) -> ("dest"=w948:refnum<vi>)
    n274 = property class="VI"(reference=w948, error in=w945) -> (error out=w946:errorcluster, "Diagram"=w947:refnum<vi>)  [unwired: 1 out]
    n275 = invoke class="TopLvlDiag" method="RemWireLooseEnds"(reference=w947, error in=w946) -> (error out=w944:errorcluster)  [unwired: 1 in, 2 out]
  }
  n276 = for {
    tunnel: w98 -> [w956] mode=indexing
    shift-right: [w950] -> w100
    shift-left: w101 -> [w955]
    # "Remove orphaned TRUE constants"
    n277 = Unbundle By Name(w956) -> ("DstDiagram"=w949:refnum<vi>)
    n278 = call <vilib>:"Traverse for GObjects.vi"("Other Refnum"=w949, "Traverse Target"=TRef_TravTarget."Other", "error in (no error)"=w955, "Class Name"="BooleanConstant") -> ("error out"=w952:errorcluster, "References"=w951:refnum<vi>[])  [unwired: 4 in, 2 out]
    n279 = for {
      shift-right: [w957] -> w950
      shift-left: w952 -> [w970]
      tunnel: w951 -> [w969] mode=indexing
      w968 = refnum<vi> refnum  # BooleanConstant
      n280 = To More Specific Class(target class=w968, reference=w969, error in=w970) -> (specific class reference=w967:refnum<vi>, error out=w966:errorcluster)
      n281 = property class="BoolCnst"(reference=w967, error in=w966) -> (reference out=w965:refnum<vi>, error out=w959:errorcluster, "Value"=w964:variant)
      n282 = Variant To Data(type=FALSE, Variant=w964) -> (data=w960:bool)  [unwired: 1 in, 1 out]
      n283 = property class="BoolCnst"(reference=w965, error in=w959) -> (reference out=w961:refnum<vi>, error out=w962:errorcluster, "Terminal.Wire.Width"=w958:u32)
      n284 = case shown="Error .." w962 {
        selector: w962 -> [w971 _]
        tunnel: w961 -> [_ w974]
        tunnel: w960 -> [_ w975]
        tunnel: [w971 w972] -> w957
        tunnel: w959 -> [_ w973]
        tunnel: w958 -> [_ _]
        frame No Error {
          # "not orphaned - do nothing"
        }
        frame Error {
          # "is orphaned - delete if TRUE"
          n285 = case shown="True" w975 {
            tunnel: w973 -> [w976 w978]
            tunnel: w974 -> [_ w979]
            tunnel: [w976 w977] -> w972
            frame False {
            }
            frame True {
              n286 = invoke class="BoolCnst" method="Delete"(reference=w979, error in=w978) -> (error out=w977:errorcluster)  [unwired: 1 in, 2 out]
            }
          }
        }
      }
    }
  }
  n287 = for {
    shift-right: [w980] -> w96
    shift-left: w100 -> [w982]
    tunnel: w99 -> [w983] mode=indexing
    # "Save the Destination VIs"
    n288 = Unbundle By Name(w983) -> ("dest"=w981:refnum<vi>)
    n289 = invoke class="VI" method="Save.Instrument"(reference=w981, error in=w982) -> (error out=w980:errorcluster)  [unwired: 4 in, 5 out]
  }
  n290 = property class="Library"(reference=w95, error in=w96) -> (error out=w79:errorcluster, "Path"=w89:path)  [unwired: 1 out]
  n291 = Strip Path(path=w89) -> (stripped path=w85:path)  [unwired: 1 out]
  n292 = invoke class="ProjectItem" method="Delete"(reference=w94, error in=w79) -> (error out=w82:errorcluster)  [unwired: 1 in, 2 out]
  n293 = Delete(path (use dialog)=w85, entire hierarchy (F)=TRUE, error in=w82) -> (error out=w81:errorcluster)  [unwired: 2 in, 2 out]
  n294 = property class="Library"(reference=w86, error in=w81) -> (error out=w68:errorcluster, "Path"=w84:path)  [unwired: 1 out]
  n295 = invoke class="ProjectItem" method="Delete"(reference=w87, error in=w68) -> (error out=w88:errorcluster)  [unwired: 1 in, 2 out]
  n296 = invoke class="Project" method="Save"(reference=w92, error in=w88) -> (reference out=w91:refnum<vi>, error out=w90:errorcluster)  [unwired: 2 in, 2 out]
  n297 = invoke class="Project" method="Close"(reference=w91, error in=w90) -> (error out=w80:errorcluster)  [unwired: 1 in, 2 out]
  n298 = invoke class="App" method="Library.Open"(error in=w80, "path"=w84) -> (error out=w43:errorcluster, "Open Library"=w48:refnum<vi>)  [unwired: 2 in, 2 out]
  n299 = local read "Source server name"() -> (w51:string)
  n300 = Strip Path(path=w84) -> (stripped path=w39:path)  [unwired: 1 out]
  n301 = Concatenate Strings(w51, ".lvlib" ("string")) -> (w41:string)
  n302 = Create Folder(path (use dialog)=w85, error in=w43) -> (error out=w42:errorcluster)  [unwired: 1 in, 2 out]
  n303 = invoke class="Library" method="Save a Copy"(reference=w48, error in=w42, "Path"=w85, "New Name"=w41) -> (reference out=w47:refnum<vi>, error out=w46:errorcluster, "New Lib Path"=w40:path)  [unwired: 2 in, 3 out]
  n304 = Close Reference(reference=w47, error in (no error)=w46) -> (error out=w45:errorcluster)
  n305 = Delete(path (use dialog)=w39, entire hierarchy (F)=TRUE, error in=w45) -> (error out=w44:errorcluster)  [unwired: 2 in, 2 out]
  n306 = local read "Project path"() -> (w61:path)
  n307 = invoke class="App" method="Project.Open"(error in=w44, "Path"=w61) -> (error out=w67:errorcluster, "Project:Open"=w62:refnum<vi>)  [unwired: 2 in, 2 out]
  n308 = local read "target name"() -> (w60:string)
  n309 = property class="Project"(reference=w62, error in=w67) -> (reference out=w53:refnum<vi>, error out=w65:errorcluster, "Targets"=w66:refnum<vi>[])
  n310 = for {
    tunnel: w66 -> [w994] mode=indexing
    shift-right: [w985] -> w59
    shift-left: w65 -> [w995]
    tunnel: w60 -> [w991]
    shift-right: [w984] -> _
    shift-left: FALSE -> [w989]
    shift-right: [w987] -> w58
    shift-left: refnum<vi> refnum ("reference out") -> [w988]
    # "Get Target Item Reference"
    n311 = property class="TargetItem"(reference=w994, error in=w995) -> (reference out=w986:refnum<vi>, error out=w990:errorcluster, "Name"=w993:string)
    n312 = Equal?(x=w993, y=w991) -> (x = y?=w992:bool)
    n313 = case shown="True" w992 {
      selector: w992 -> [_ w1001]
      tunnel: w990 -> [w999 w1002]
      tunnel: w989 -> [w996 _]
      tunnel: w988 -> [w997 _]
      tunnel: [w997 w1003] -> w987
      tunnel: w986 -> [w998 w1003]
      tunnel: [w1000 w1002] -> w985
      tunnel: [w996 w1001] -> w984
      frame False {
        n314 = Close Reference(reference=w998, error in (no error)=w999) -> (error out=w1000:errorcluster)
      }
      frame True {
      }
    }
  }
  n315 = invoke class="TargetItem" method="AddItem"(reference=w58, error in=w59, "Name"=w51, "Path"=path "", "Type"="Folder") -> (error out=w50:errorcluster, "AddItem"=w54:refnum<vi>)  [unwired: 1 in, 4 out]
  n316 = invoke class="ProjectItem" method="AddItem"(reference=w54, error in=w50, "Name"=w41, "Path"=w40, "Type"="Library") -> (error out=w49:errorcluster)  [unwired: 1 in, 5 out]
  n317 = invoke class="Project" method="Save"(reference=w53, error in=w49) -> (error out=→"error out":errorcluster)  [unwired: 2 in, 3 out]
